vi "Configure SBUS Normal.vi"(7 "Enable Display (T: Enable)":bool=TRUE, 8 "error in (no error)":errorcluster, 9 "Decode Mode (0: IIC)":i32(ring)=1 items=["IIC", "SPI", "CAN"], 10 "Channel (1: Serial Bus 1)":i32(ring)=1 items=["Serial Bus 1"=1, "Serial Bus 2"=2, "Serial Bus 3"=3, "Serial Bus 4"=4], 11 "VISA resource name":refnum<visa-resource-name>) -> (0 "error out":errorcluster, 3 "VISA resource name out":refnum<visa-resource-name>)   [LabVIEW 2020, in "Agilent 90000 Series.lvlib"]
doc: "Configures the display and decode mode for the serial bus.\n\n<B>Note:</B>\nThis VI is only valid when a serial decode option has been licensed."
uses:
  Agilent 90000 Series.lvlib
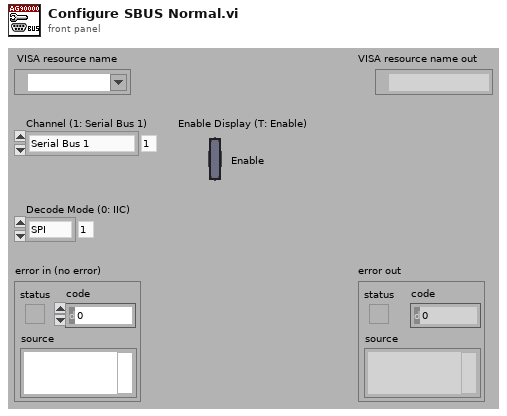
[diagram p1: front panel]
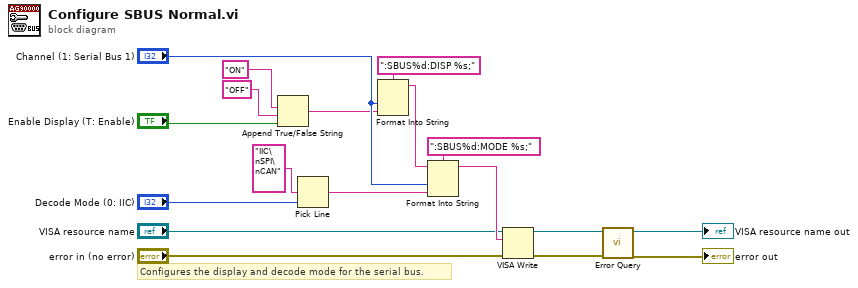
[diagram p0: block diagram]
diagram:
  # "Configures the display and decode mode for the serial bus."
  n1 = Append True/False String(1:"Enable Display (T: Enable)", 2:"OFF", 3:"ON") -> (0:w13:string)  [unwired: 1 out]
  n2 = Pick Line(multi-line string="IIC\nSPI\nCAN", line index="Decode Mode (0: IIC)") -> (output string=w8:string)  [unwired: 1 out]
  n3 = Format Into String(format string=":SBUS%d:DISP %s;", "Channel (1: Serial Bus 1)", w13) -> (resulting string=w10:string)  [unwired: 2 in, 1 out]
  n4 = Format Into String(format string=":SBUS%d:MODE %s;", initial string=w10, "Channel (1: Serial Bus 1)", w8) -> (resulting string=w7:string)  [unwired: 1 in, 1 out]
  n5 = VISA Write(VISA resource name="VISA resource name", write buffer=w7, error in (no error)="error in (no error)") -> (VISA resource name out=w4:refnum<visa-resource-name>, error out=w3:errorcluster)  [unwired: 1 out]
  n6 = call "Error Query.vi"("error in (no error)"=w3, "VISA resource name"=w4) -> ("error out"=→"error out":errorcluster, "VISA resource name out"=→"VISA resource name out":refnum<visa-resource-name>)  [unwired: 8 out]
